vi "Vertical Grid Lines.vi"(8 "error in (no error)":errorcluster, 10 "Segment":i32, 11 "No. of veritcal lines":i32) -> (0 "error out":errorcluster, 3 "Length":i32)   [LabVIEW 2017]
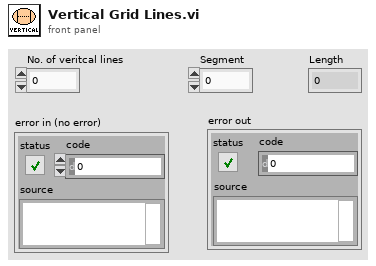
[diagram p1: front panel]
types:
  T1 = enum16{"Full", "Half", "Quarter", "Eighth", "Sixteenth"}
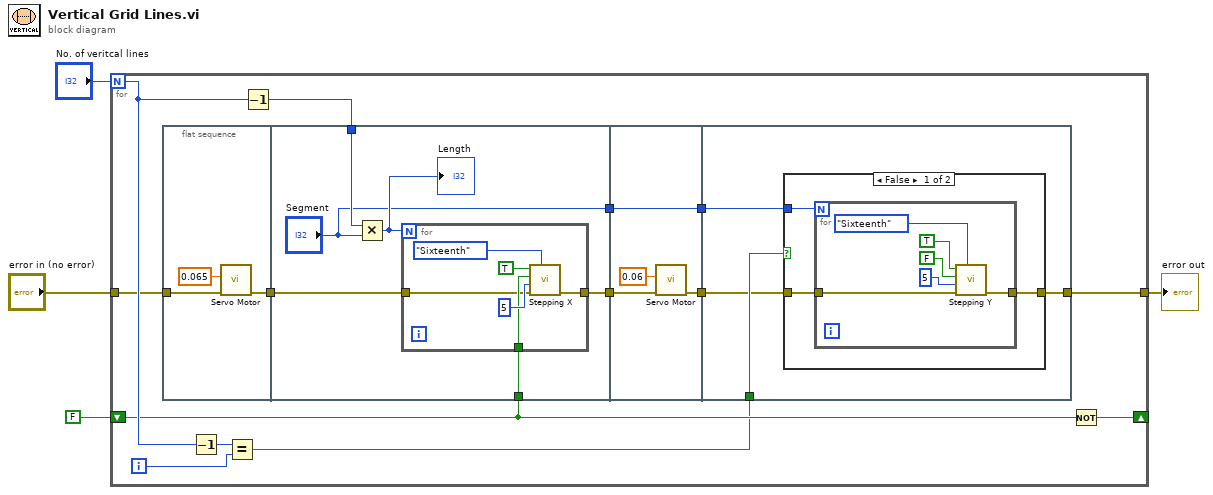
[diagram p0: block diagram]
diagram:
  n1 = for {
    N: "No. of veritcal lines" -> [w15]
    shift-right: [w18] -> _
    shift-left: FALSE -> [w12]
    tunnel: "error in (no error)" -> [w7]
    tunnel: [w6] -> w2
    i -> [w16]
    n2 = flat-sequence {
      tunnel: [w20] -> w10
      tunnel: w7 -> [w19]
      tunnel: w5 -> [w27]
      tunnel: ["Segment"] -> w14
      tunnel: w12 -> [w24]
      tunnel: w10 -> [w23]
      tunnel: [w22] -> w9
      tunnel: w14 -> [w36]
      tunnel: [w36] -> w13
      tunnel: w9 -> [w35]
      tunnel: [w34] -> w8
      tunnel: w13 -> [w41]
      tunnel: w11 -> [w40]
      tunnel: w8 -> [w39]
      tunnel: [w38] -> w6
      frame #0 {
        n3 = call "Servo Motor.vi"("error in (no error)"=w19, "Duty Cycle"=0.065) -> ("error out"=w20:errorcluster)  [unwired: 8 in, 1 out]
      }
      frame #1 {
        n4 = Multiply(x=w27, y="Segment") -> (x*y=w26:i32)
        "Length" <- w26
        n5 = for {
          N: w26 -> [_]
          tunnel: w24 -> [w30]
          tunnel: w23 -> [w29]
          tunnel: [w28] -> w22
          n6 = call "Stepping X.vi"("Microstep size"=T1."Sixteenth", "error in (no error)"=w29, "Speed"=u32 5, "Direction"=w30, "Enable"=TRUE) -> ("error out"=w28:errorcluster)  [unwired: 6 in]
        }
      }
      frame #2 {
        n7 = call "Servo Motor.vi"("error in (no error)"=w35, "Duty Cycle"=0.06) -> ("error out"=w34:errorcluster)  [unwired: 8 in, 1 out]
      }
      frame #3 {
        n8 = case shown="False" w40 {
          tunnel: w41 -> [w44 _]
          tunnel: w39 -> [w43 w51]
          tunnel: [w42 w51] -> w38
          frame False {
            n9 = for {
              N: w44 -> [_]
              tunnel: w43 -> [w46]
              tunnel: [w45] -> w42
              n10 = call "Stepping Y.vi"("Microstep size"=T1."Sixteenth", "error in (no error)"=w46, "Speed"=u32 5, "Direction"=FALSE, "Enable"=TRUE) -> ("error out"=w45:errorcluster)  [unwired: 6 in]
            }
          }
          frame True {
          }
        }
      }
    }
    n11 = Decrement(x=w15) -> (x-1=w17:i32)
    n12 = Equal?(x=w17, y=w16) -> (x = y?=w11:bool)
    n13 = Decrement(x=w15) -> (x-1=w5:i32)
    n14 = Not(x=w12) -> (.not. x?=w18:bool)
  }
  "error out" <- w2
